vi "XYStage Sweep Control.vi"(6 "Dirrection in":T1, 8 "Y Count":i32, 9 "X Count":i32, 10 "Y Index in":i32, 11 "X Index in":i32) -> (0 "New Row?":bool, 1 "Next?":bool, 2 "Y Index out":i32, 3 "X Index out":i32, 4 "Dirrection out":T1)   [LabVIEW 2017, in "Measurement.PhotocurrentMapping.lvclass"]
uses:
  Measurement.PhotocurrentMapping.lvclass
  Typedefs/Scanning Direction--Enum.ctl
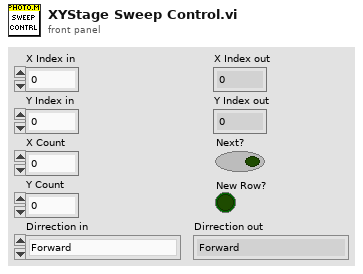
[diagram p1: front panel]
types:
  T1 = typedef "Measurement.PhotocurrentMapping.lvclass/Scanning Direction--Enum.ctl" = enum16{"Forward", "Backward"}
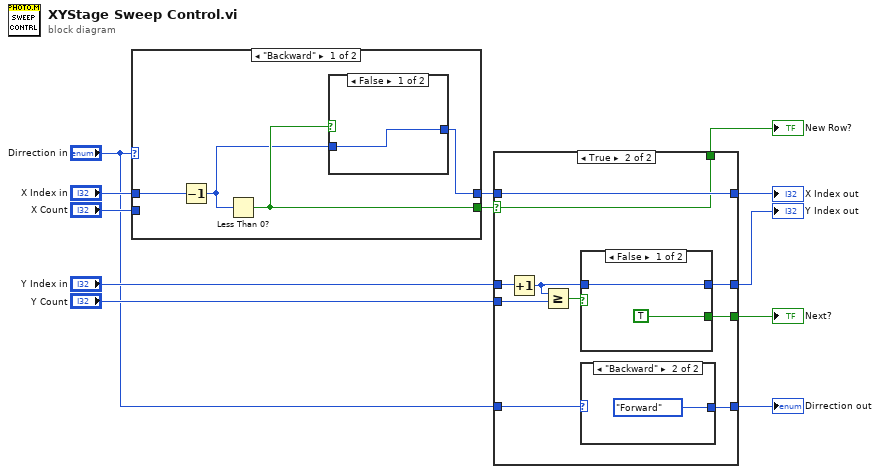
[diagram p0: block diagram]
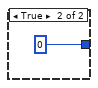
[diagram p2: hidden frame]
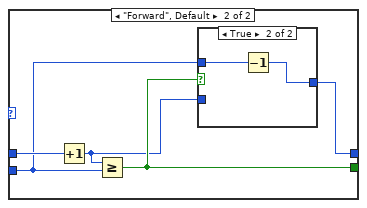
[diagram p3: hidden frame]
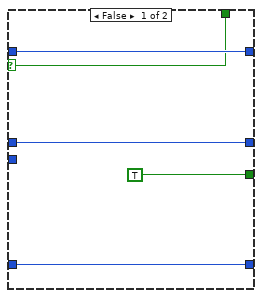
[diagram p5: hidden frame]
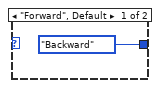
[diagram p6: hidden frame]
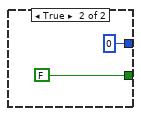
[diagram p7: hidden frame]
diagram:
  n1 = case shown="\"Backward\"" "Dirrection in" {
    tunnel: [w14 w19] -> w9
    tunnel: [w15 w22] -> w6
    tunnel: "X Count" -> [_ w20]
    tunnel: "X Index in" -> [w16 w23]
    frame "Backward" {
      n2 = Decrement(x=w16) -> (x-1=w13:i32)
      n3 = Less Than 0?(x=w13) -> (x < 0?=w15:bool)
      n4 = case shown="False" w15 {
        tunnel: w13 -> [w17 _]
        tunnel: [w17 0] -> w14
        frame False {
        }
        frame True {
        }
      }
    }
    frame "Forward", Default {
      n5 = Increment(x=w23) -> (x+1=w21:i32)
      n6 = Greater Or Equal?(x=w21, y=w20) -> (x >= y?=w22:bool)
      n7 = case shown="True" w22 {
        tunnel: w21 -> [w24 _]
        tunnel: w20 -> [_ w26]
        tunnel: [w24 w25] -> w19
        frame False {
        }
        frame True {
          n8 = Decrement(x=w26) -> (x-1=w25:i32)
        }
      }
    }
  }
  n9 = case shown="True" w6 {
    selector: w6 -> [w27 w32]
    tunnel: "Y Index in" -> [w30 w41]
    tunnel: "Y Count" -> [_ w40]
    tunnel: w9 -> [w31 w35]
    tunnel: [w31 w35] -> w10
    tunnel: [w30 w37] -> w11
    tunnel: [TRUE w36] -> w12
    tunnel: "Dirrection in" -> [w28 w34]
    tunnel: [w28 w33] -> w2
    tunnel: [w27 w32] -> w1
    frame False {
    }
    frame True {
      n10 = Increment(x=w41) -> (x+1=w38:i32)
      n11 = Greater Or Equal?(x=w38, y=w40) -> (x >= y?=w39:bool)
      n12 = case shown="False" w39 {
        tunnel: w38 -> [w45 _]
        tunnel: [w45 0] -> w37
        tunnel: [TRUE FALSE] -> w36
        frame False {
        }
        frame True {
        }
      }
      n13 = case shown="\"Backward\"" w34 {
        tunnel: [Scanning_Direction--Enum."Backward" ("Dirrection in") Scanning_Direction--Enum."Forward" ("Dirrection in")] -> w33
        frame "Forward", Default {
        }
        frame "Backward" {
        }
      }
    }
  }
  "Next?" <- w12
  "Y Index out" <- w11
  "X Index out" <- w10
  "Dirrection out" <- w2
  "New Row?" <- w1
